vi "Conditional disabled state-Speed graph behaviour ctrl.vi"(8 "error in (no error)":errorcluster, 10 "Disabled":T1(ring)) -> (0 "error out":errorcluster)   [LabVIEW 2020]
uses:
  Patch-Vol video generator/Globals/gl_8-bit montage window ctrl refs.vi
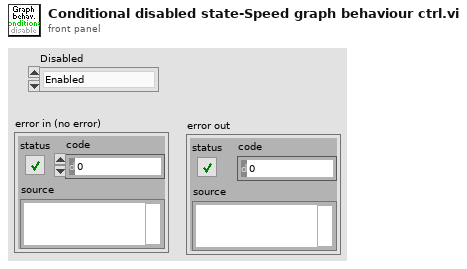
[diagram p1: front panel]
types:
  T1 = enum8{"Enabled", "Disabled", "Disabled and Grayed Out"}
  T2 = typedef "8-bit video export window ctrl refs.ctl" = cluster{"This VI":refnum<vi>, "Add speed data":refnum<vi>, "Add camera videos":refnum<vi>, "Stop button":refnum<vi>, "Camera Video Adjustments":refnum<vi>, "Microscope Image Adjustments":refnum<vi>, "Execute":refnum<vi>, "Codec":refnum<vi>, "Channel to load":refnum<vi>, "Speed graph behaviour":refnum<vi>, "Include speed graph":refnum<vi>, "Number of rows to generate":refnum<vi>, "Path":refnum<vi>}
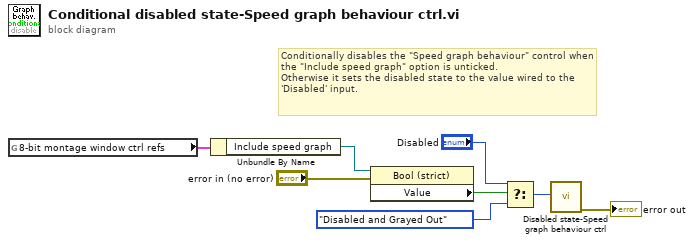
[diagram p0: block diagram]
diagram:
  # "Conditionally disables the \"Speed graph behaviour\" control when the \"Include speed graph\" option is unticked.\nOtherwise it sets the disabled state to the value wired to the 'Disabled' input."
  n1 = global read "gl_8-bit montage window ctrl refs.vi" "8-bit montage window ctrl refs"() -> (w7:T2)
  n2 = Unbundle By Name(w7) -> ("Include speed graph"=w1:refnum<vi>)
  n3 = property on="Property Node" class="Bool (strict)"(reference=w1, error in="error in (no error)") -> ("Value"=w6:bool)  [unwired: 2 out]
  n4 = Select(t="Disabled", s=w6, f=T1."Disabled and Grayed Out") -> (s? t:f=w3:T1)
  n5 = call "Disabled state-Speed graph behaviour ctrl.vi"("Disabled"=w3) -> ("error out"=→"error out":errorcluster)  [unwired: 10 in]
